vi "读取Vtemp.vi"(8 "error in":errorcluster) -> (0 "error out":errorcluster, 1 "return":i32, 2 "VTemp":u16)   [LabVIEW 2016]
panel:
  out "data out":u8[](array[numeric])
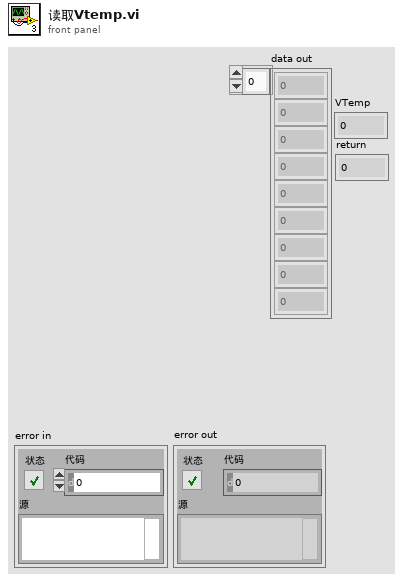
[diagram p1: front panel]
types:
  T1 = cluster{"byCmdType":u8, "bySubCmd":u8, "byPara":u8, "byAddr_h":u8, "byAddr_l":u8, "byAddr_ll":u8, "byLen_h":u8, "byLen_l":u8}
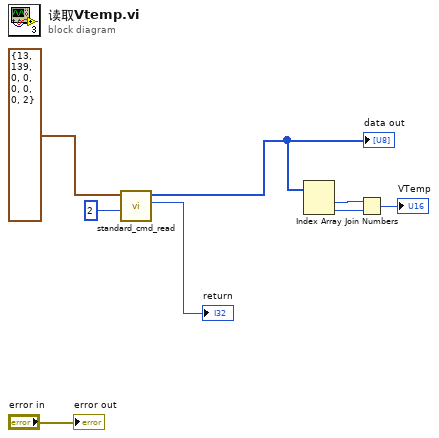
[diagram p0: block diagram]
diagram:
  n1 = call "standard_cmd_read.vi"("dwLen"=u32 2 ("dwAddr"), "cmd_std_header_t"=T1 {"byCmdType"=13, "bySubCmd"=139, "byPara"=0, "byAddr_h"=0, "byAddr_l"=0, "byAddr_ll"=0, "byLen_h"=0, "byLen_l"=2}) -> ("return"=→"return":i32, "data out"=w5:u8[])  [unwired: 8 in]
  "data out" <- w5
  n2 = Index Array(array=w5) -> (element #1=w4:u8, element #2=w3:u8)  [unwired: 2 in]
  n3 = Join Numbers(hi=w4, lo=w3) -> ((hi.lo)=→"VTemp":u16)
  "error out" <- "error in"
